vi "IMUOrientOpen.vi"(5 "Stored Cal File":string="BNO055 Cal MC P3 11-28-2015 145653", 7 "Calibrate?":bool, 8 "Status delay":i32=30, 9 "I2C Bus 2":T3=enum."I2C MXP", 10 "Placement":T8(ring)=enum."P3", 11 "Op Mode":T6(ring)=enum."NDOF") -> (0 "Bad result":bool, 2 "Cal Status":T4, 3 "I2CDevRef":T1={"DevStatus"={"status"=FALSE, "code"=0, "source"=""}, "Controller"=enum."Controller 1", "Device Address"=0, "Handle"=0, "I2C Bus"=enum."Invalid"} {"Device Address" format="%.0x"})   [LabVIEW 2014]
uses:
  <vilib>/Rock Robotics/SystemInterfaces/i2clib/i2c_bus.ctl
  Setup State.ctl
  <vilib>/Rock Robotics/WPI/I2C/WPI_I2CDevRef.ctl
  <vilib>/Rock Robotics/SystemInterfaces/Typedef/FPGA_TypedefDigitalModule.ctl
panel:
  out "Bad ct":i32
  out "SC ct":i32
  out "S":T5
  out "G":T5
  out "A":T5
  out "M":T5
  out "Bad result":bool
  out "Fusion":bool
  out "Fusion ct":i32
  out "Reset ct":i32
  out "Occupant":u8[](array[numeric]) format="%02x"
  out "Setup ct":i32
  out "Setup State":T7
  # "Manual Cal\nCalibration Status Indicator"
  # "Diagnostics"
  # "These controls/indicators are non-operational / they are here as example documentation only."
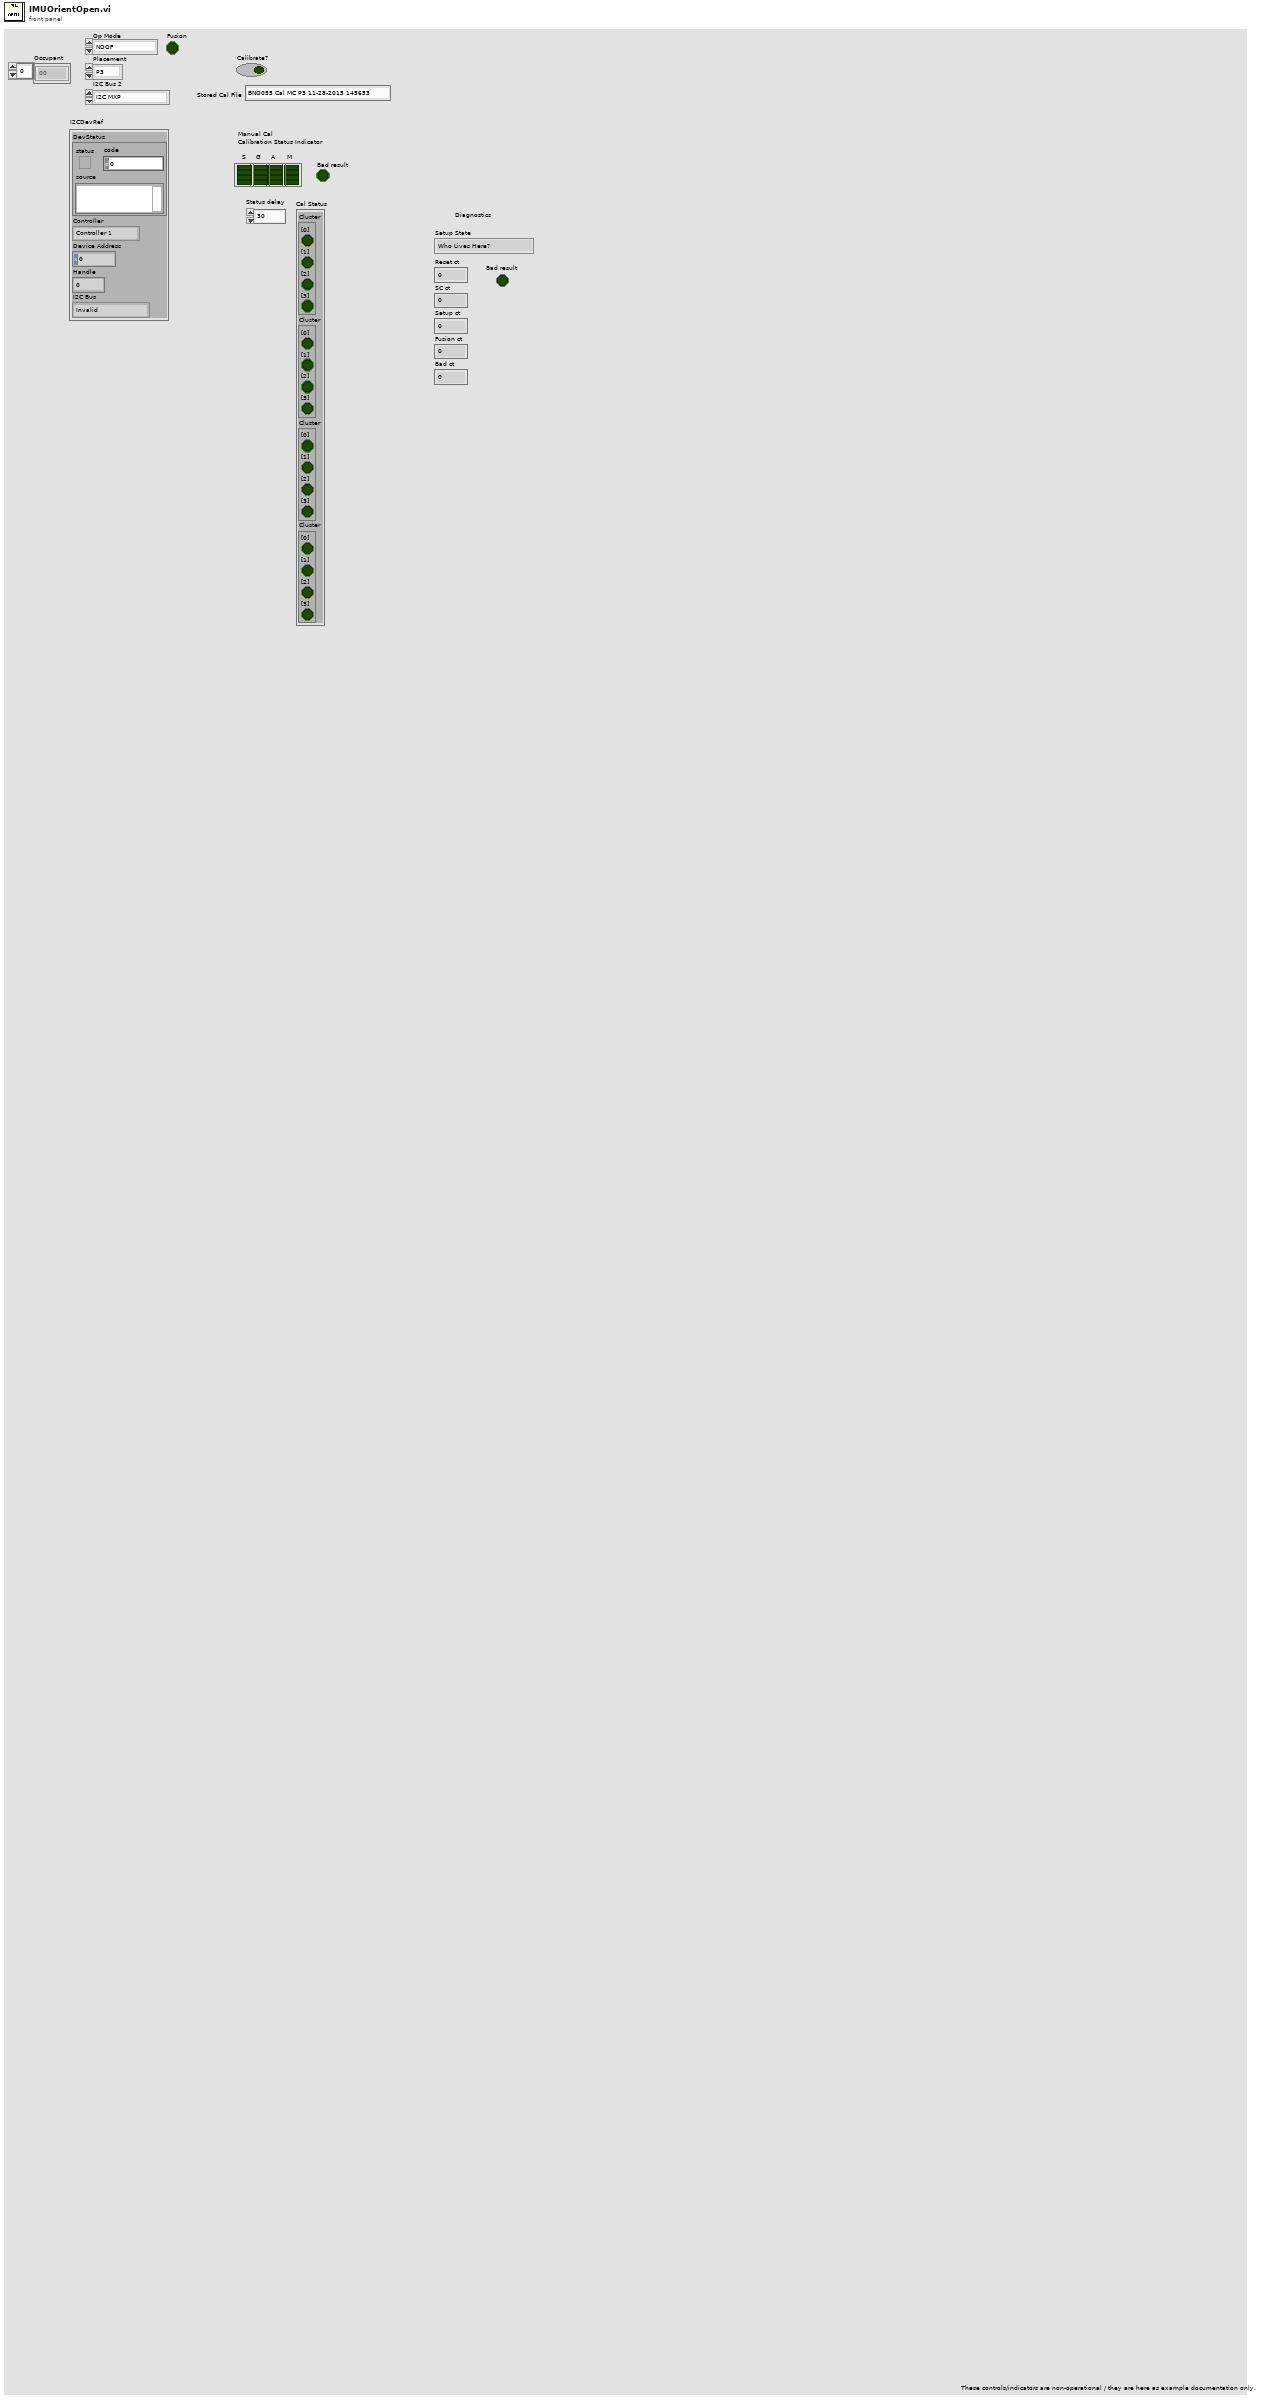
[diagram p1: front panel]
types:
  T1 = typedef "WPI_I2CDevRef.ctl" = cluster{"DevStatus":errorcluster, "Controller":T2, "Device Address":u8, "Handle":i32, "I2C Bus":T3}
  T2 = typedef "FPGA_TypedefDigitalModule.ctl" = enum16{"Controller 1"}
  T3 = typedef "i2c_bus.ctl" = enum16{"I2C On-Board", "I2C MXP", "Invalid"}
  T4 = cluster{"Cluster":cluster{"[0]":bool, "[1]":bool, "[2]":bool, "[3]":bool}, "Cluster":cluster{"[0]":bool, "[1]":bool, "[2]":bool, "[3]":bool}, "Cluster":cluster{"[0]":bool, "[1]":bool, "[2]":bool, "[3]":bool}, "Cluster":cluster{"[0]":bool, "[1]":bool, "[2]":bool, "[3]":bool}}
  T5 = cluster{"Boolean":bool, "Boolean 2":bool, "Boolean 3":bool, "Boolean 4":bool}
  T6 = enum8{"ConfigMode", "AccOnly", "MagOnly", "GyroOnly", "AccMag", "AccGyro", "MagGyro", "AMG", "IMU", "Compass", "M4G", "NDOF_FMC_OFF", "NDOF"}
  T7 = typedef "Setup State.ctl" = enum16{"Who Lives Here?", "Config Mode", "Page 0", "Reset", "Units, Xtal, & Placement", "Fusion Mode", "Pre Calibration", "Error Check", "Manual Cal", "Save Cal", "Restore Cal", "Cal Status", "Idle"}
  T8 = enum32{"P0", "P1", "P2", "P3", "P4", "P5", "P6", "P7"}
  T9 = enum16{"open", "open or create", "create or replace", "create", "open (read-only)"}
  T10 = enum8{"ConfigMode", "AccOnly", "MagOnly", "GyroOnly", "AccMag", "AccGyro", "MagGyro", "AMG", "IMU", "Compass", "M4G", "NDOF_FMC_OFF", "NDOF"}[]
  T11 = cluster{"[0]":bool, "[1]":bool, "[2]":bool, "[3]":bool}
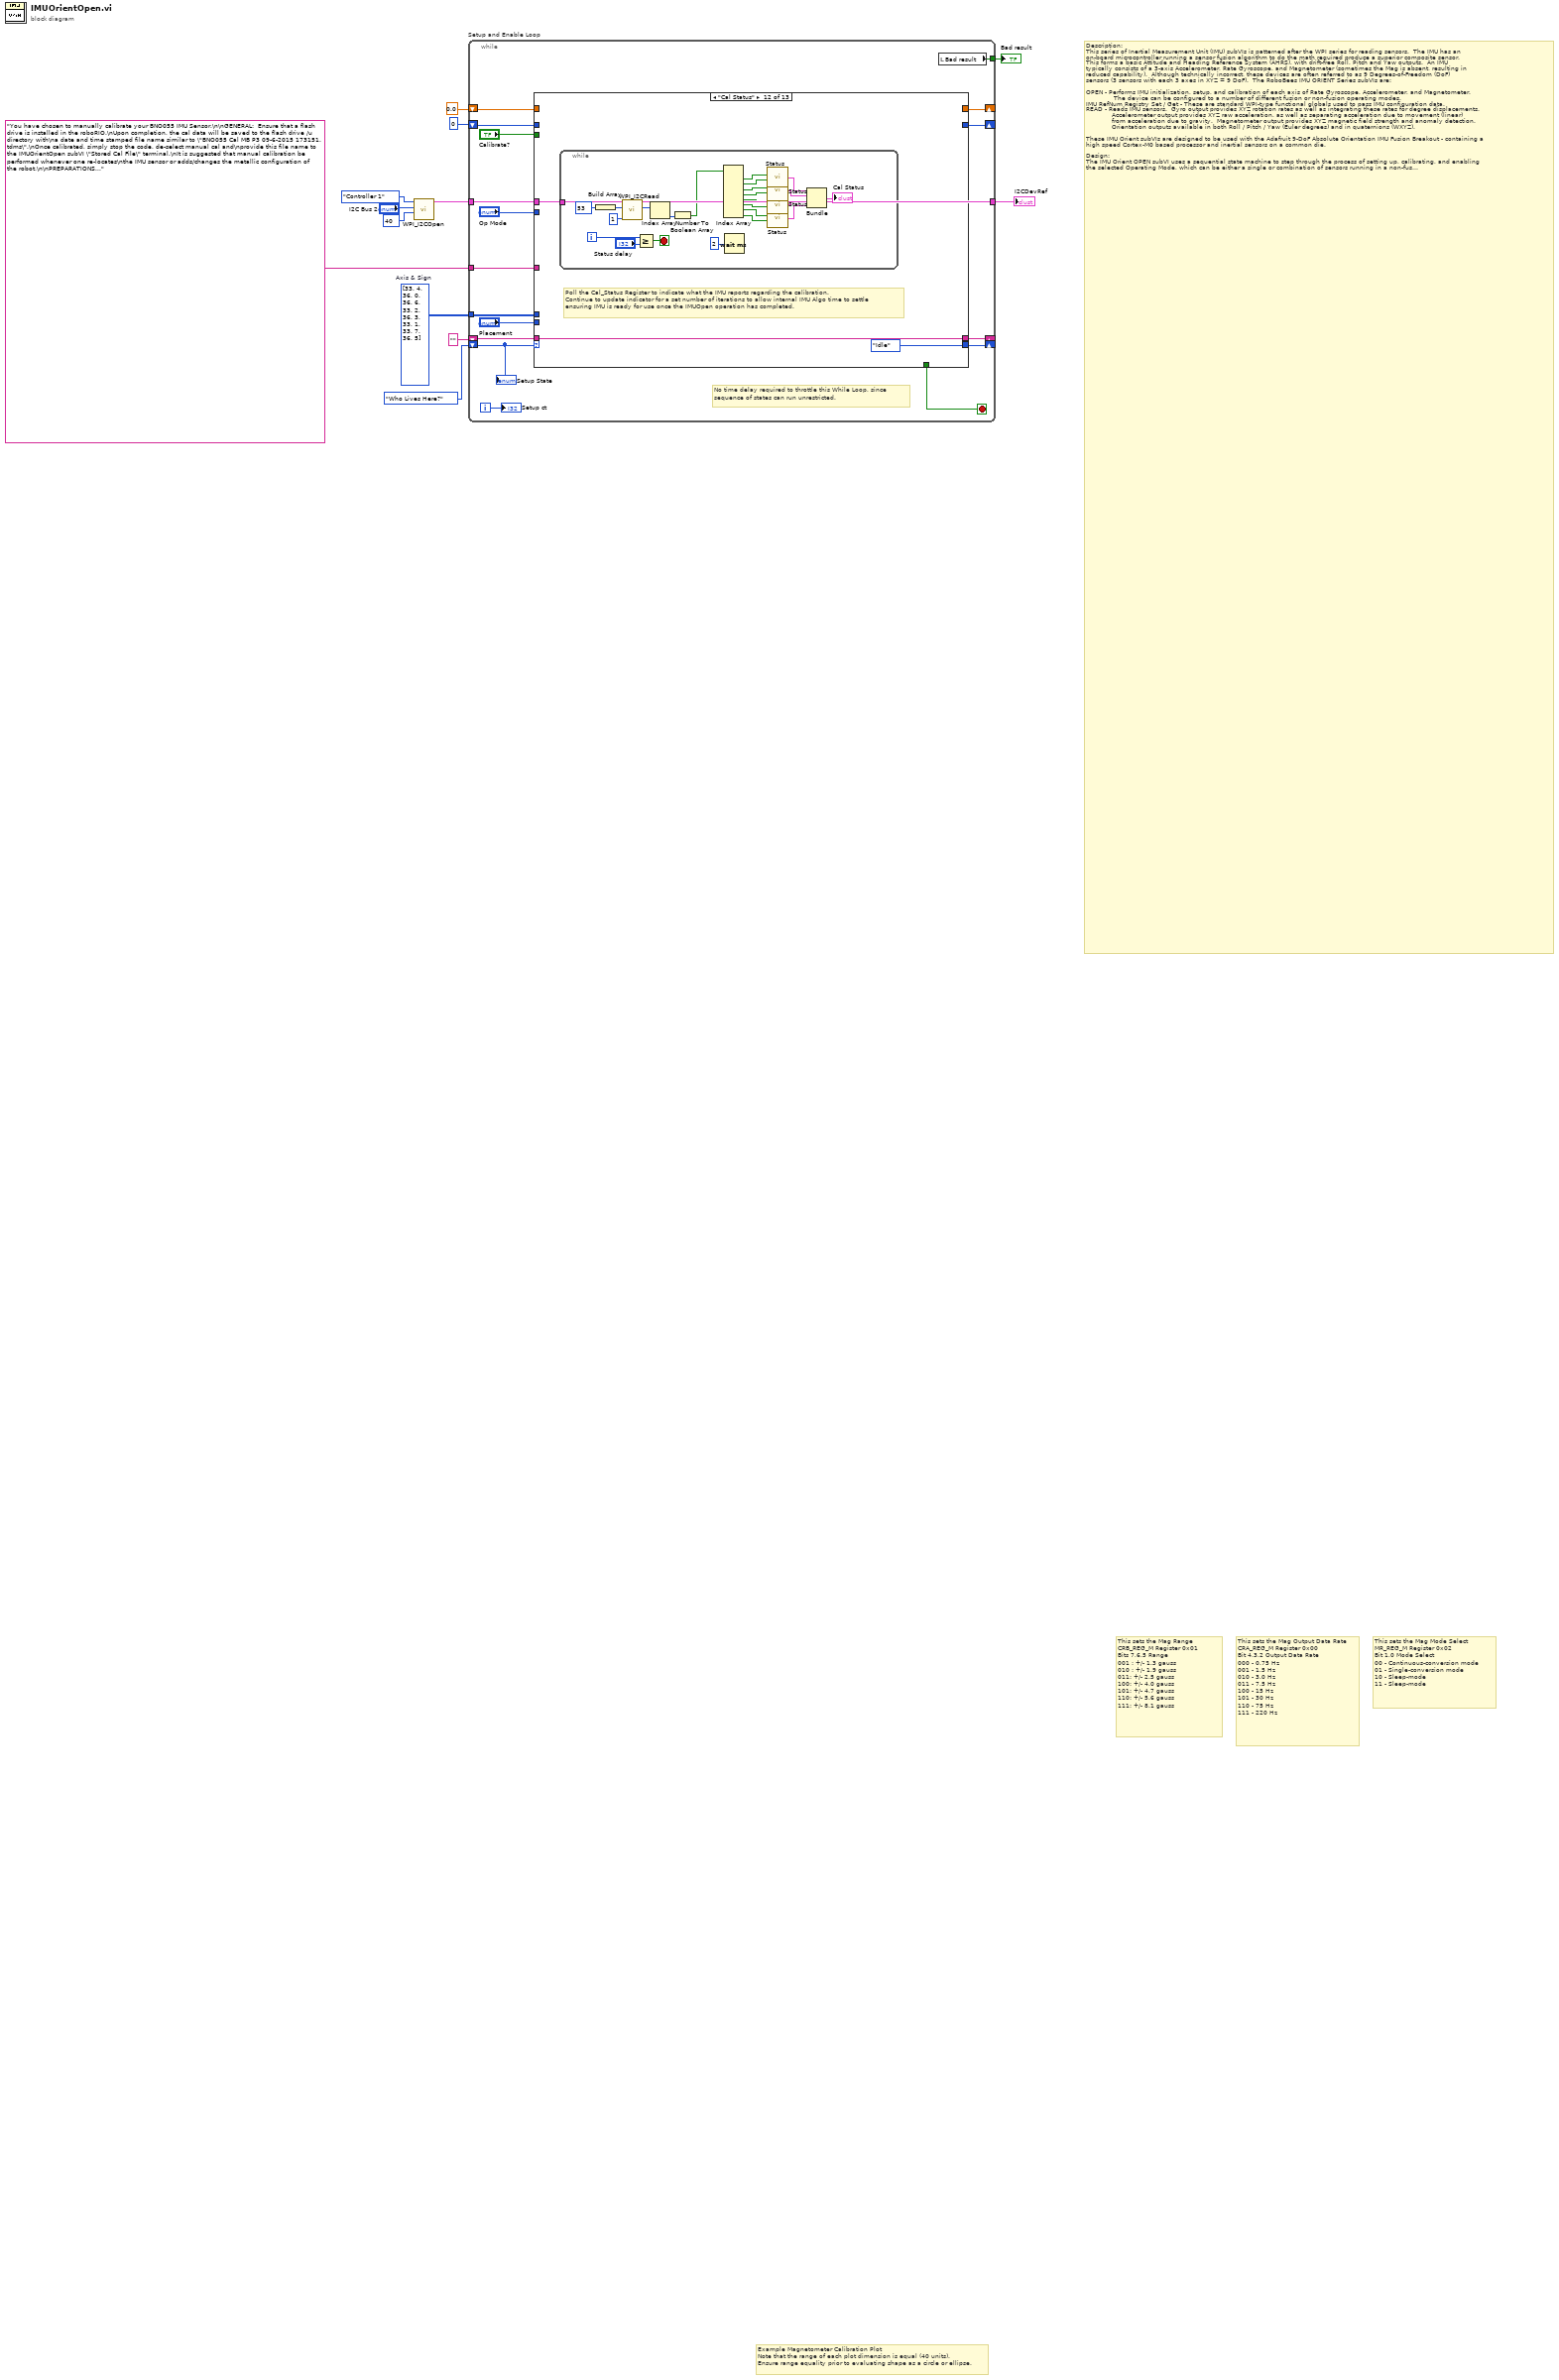
[diagram p0: block diagram]
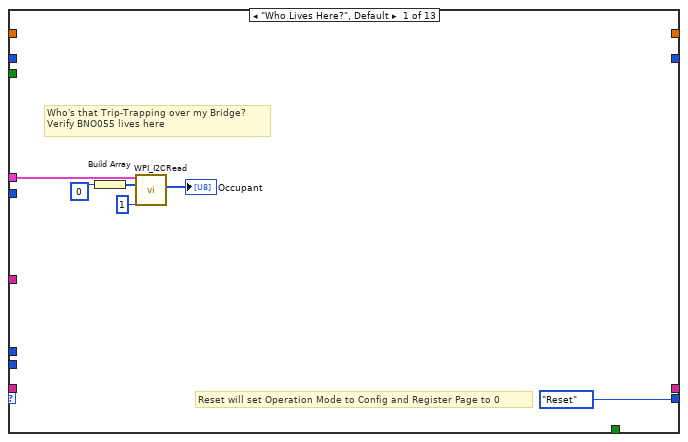
[diagram p2: hidden frame]
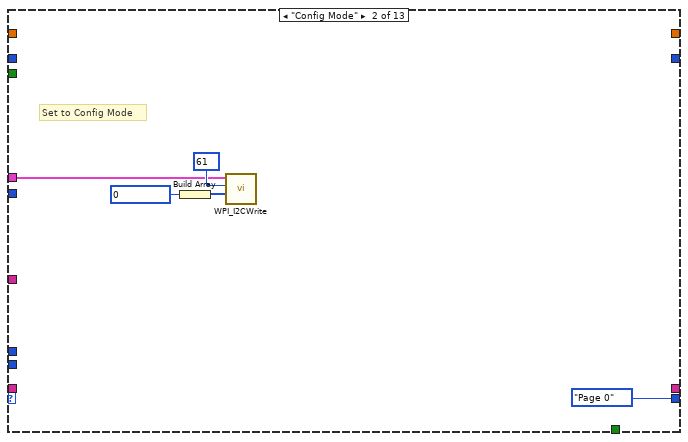
[diagram p3: hidden frame]
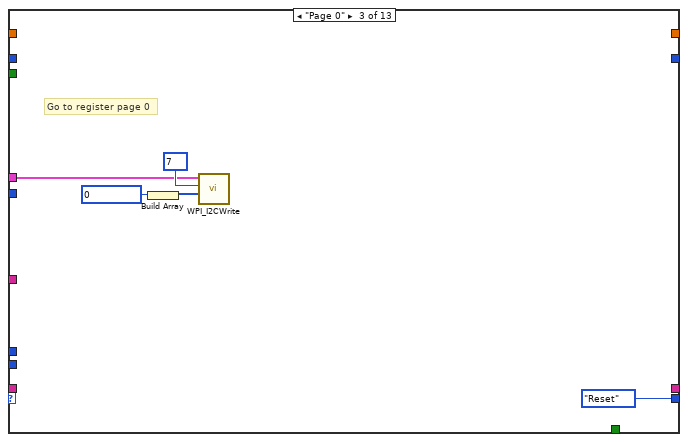
[diagram p4: hidden frame]
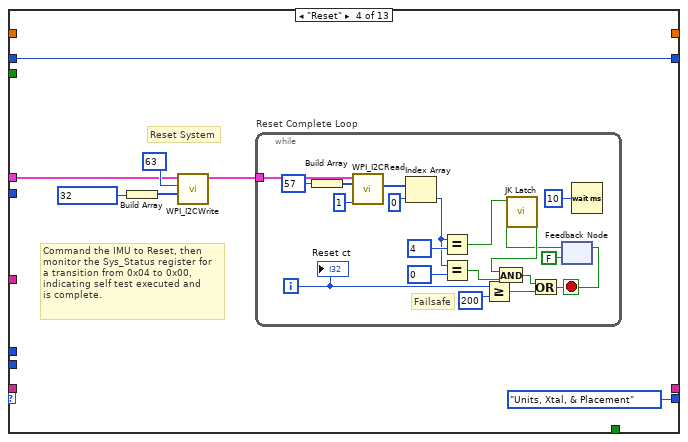
[diagram p5: hidden frame]
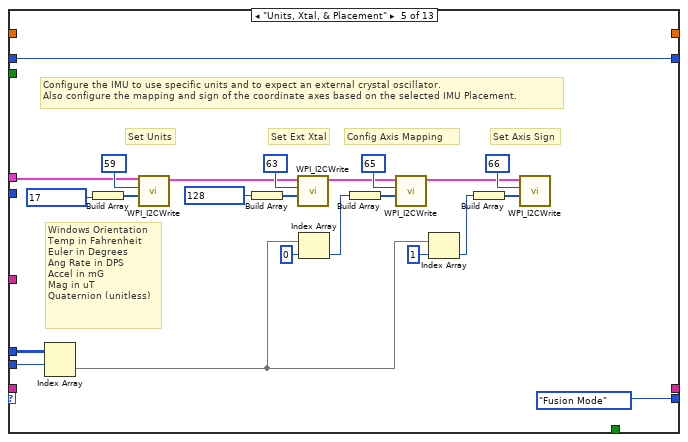
[diagram p6: hidden frame]
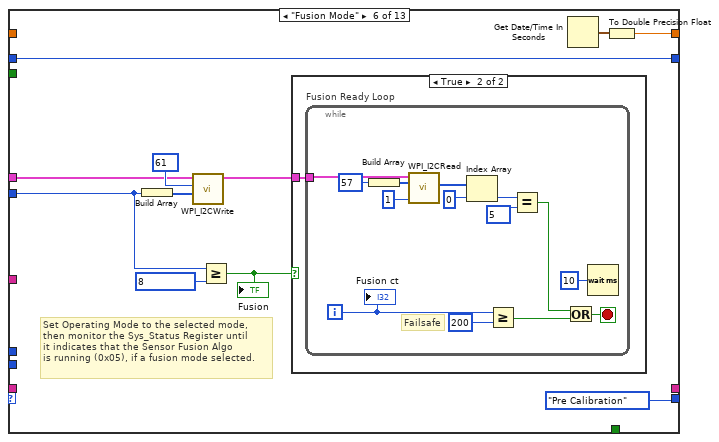
[diagram p7: hidden frame]
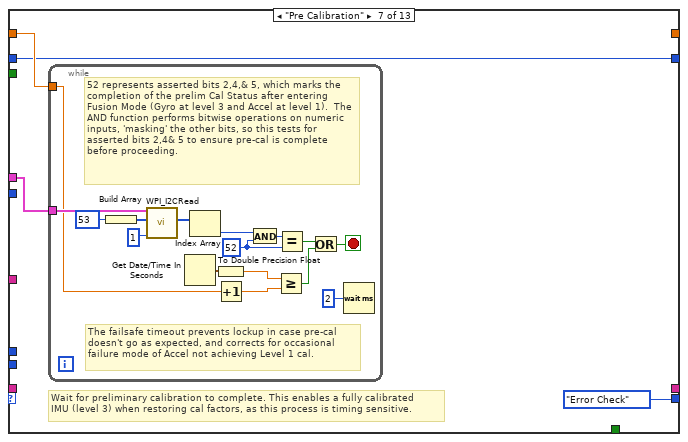
[diagram p9: hidden frame]
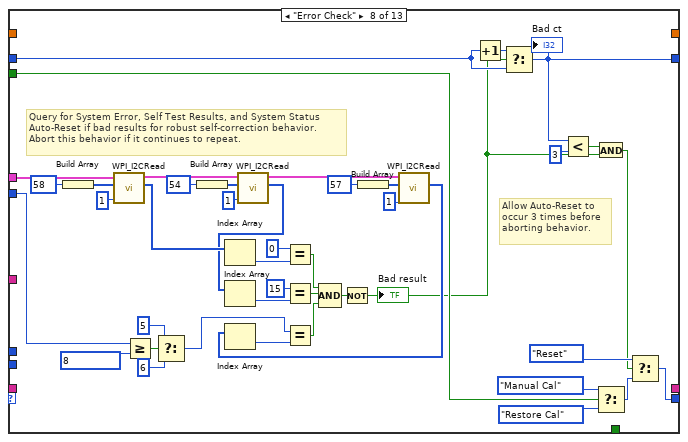
[diagram p10: hidden frame]
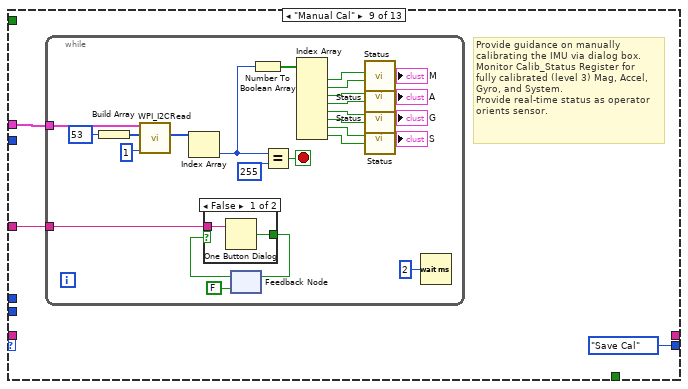
[diagram p11: hidden frame]
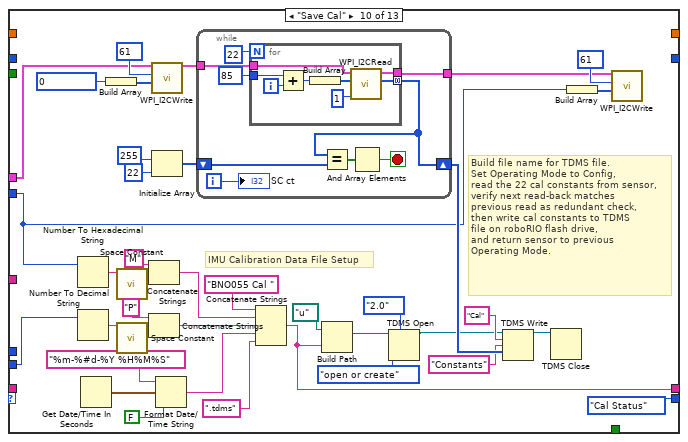
[diagram p13: hidden frame]
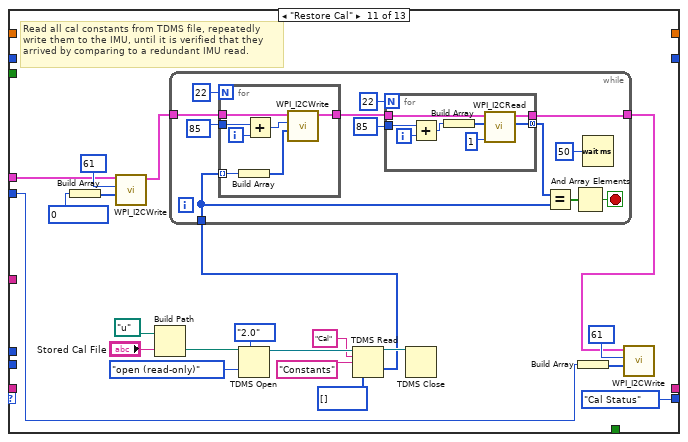
[diagram p14: hidden frame]
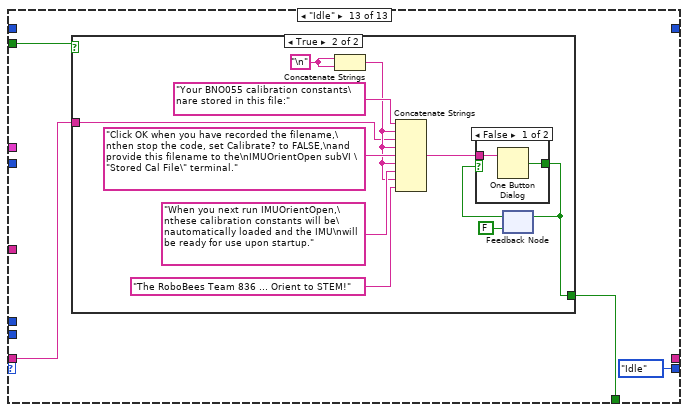
[diagram p15: hidden frame]
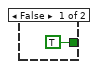
[diagram p16: hidden frame]
diagram:
  w8 = u8[][] [[33, 4], [36, 0], [36, 6], [33, 2], [36, 3], [33, 1], [33, 7], [36, 5]]  # Axis & Sign
  # "Description:\nThis series of Inertial Measurement Unit (IMU) subVIs is patterned after the WPI series for reading sensors.  The IMU has an\non-board microcontroller running a sensor fusion algorithm to do the math required produce a superior composite sensor.\nThis forms a basic Attitude and Heading Reference System (AHRS), with drift-free Roll, Pitch and Yaw outputs.  An IMU\ntypically consists of a 3-axis Accelerometer, Rate Gyroscope, and Magnetometer (sometimes the Mag is absent, resulting in\nreduced capability).  Although technically incorrect, these devices are often referred to as 9 Degrees-of-Freedom (DoF)\nsensors (3 sensors with each 3 axes in XYZ = 9 DoF).  The RoboBees IMU ORIENT Series subVIs are:\n\nOPEN - Performs IMU initialization, setup, and calibration of each axis of Rate Gyroscope, Accelerometer, and Magnetometer.\n              The device can be configured to a number of different fusion or non-fusion operating modes.\nIMU RefNum Registry Set / Get - These are standard WPI-type functional globals used to pass IMU configuration data.\nREAD - Reads IMU sensors.  Gyro output provides XYZ rotation rates as well as integrating these rates for degree displacements.\n             Accelerometer output provides XYZ raw acceleration, as well as separating acceleration due to movement (linear)\n             from acceleration due to gravity.  Magnetometer output provides XYZ magnetic field strength and anomaly detection.\n             Orientation outputs available in both Roll / Pitch / Yaw (Euler degrees) and in quaternions (WXYZ).\n\nThese IMU Orient subVIs are designed to be used with the Adafruit 9-DoF Absolute Orientation IMU Fusion Breakout - containing a\nhigh speed Cortex-M0 based processor and inertial sensors on a common die.\n\nDesign:\nThe IMU Orient OPEN subVI uses a sequential state machine to step through the process of setting up, calibrating, and enabling\nthe selected Operating Mode, which can be either a single or combination of sensors running in a non-fusion mode, or one of\nseveral fusion operating modes.\n\nThe IMU breakout board from Adafruit.com has a single I2C bus for communication.  The sensor I2C Address (in hex) and\nrespective data sheets for I2C register references are:\n\nI2C Address  -  Data Sheet Reference\n       0x28        -  https://ae-bst.resource.bosch.com/media/products/dokumente/bno055/BST_BNO055_DS000_13.pdf\n\nNote: The Adafruit website links to an older version of the BNO055 spec sheet (ver 1.2).  The Bosch site will maintain the latest\nversion.  The link above is the latest revision (ver 1.3) as of January 2016 (released August 2015).   This is a highly sophisticated\nsensor, with many control options, so it is recommended that one review the spec sheet to understand all its capabilities.\n\nSome design effort was expended in an attempt to ensure high reliability of operation.  Data transfer between the sensor cal registers\nand the required flash drive (where cal constants are stored during power down periods) is redundantly verified to be successful.  (Testing\nindicated this to be necessary.)  Upon initialization, if the sensor fails its internal self test, the code will attempt to reset the sensor.\nThis will only occur three times to avoid an infinite loop, which might otherwise prevent a robot from executing operations code.\n\nCalibration:\nRaw readings from an IMU are not very useful until they are conditioned by carefully determined calibration parameters.  One of\nthe key differences between this IMU and others, such as the one discussed here: \n\n                                                         http://www.chiefdelphi.com/forums/showthread.php?t=131823 \n\nis that this BNO055 contains an integrated microcontroller, running a sensor fusion algorithm, which is designed to constantly\nself-calibrate in real-time, after an initial calibration process has occurred.  So, unlike other IMUs that require interface code, this\nIMU really only requires code to trigger the on-board calibration code.  This makes the code for the sensor READ operations simple,\nand the complex code integration requirement associated only with the sensor OPEN (although one only has to trigger the on-board\ncal process, doing this reliably and providing functionality to store/reload the results still drives code sophistication requirements).\n\nOnce the state machine has initialized the sensor, a user-selected control is referenced to either initiate the sensor's embedded\ncal process or read previously stored calibration constants from a file.  [Note: this vi expects a flash drive to be installed in one\nof the roboRIOs USB ports for cal file storage/retrieval].   A dialog box is used to instruct the user on the sensor movements required\nfor calibration, and a Calibration Status Indicator is provided on this vi's front panel to provide feedback and track progress.   Once\ncal is complete, the filename containing the cal constants is displayed.  De-selecting the cal control and providing the cal filename\nto this vi enables the sensor to open in a ready-for-use state.\n\nThe cal filename will contain the Operating Mode, Placement (sensor orientation), and a timestamp to help distinguish one file\nfrom another.  The Op Mode and Placement are included as there is some indication in testing that one should not expect the cal\nto be correct when these parameters differ between cal and use.\n\nVI Properties:\nExecution Reentrancy is set to Non Reentrant Execution\n\nImplementation:\nIt is recommended that the MXP I2C Interface is used, rather than the On-Board I2C Interface, as the latter can generate glitches from\nLo/Hi byte pairing failures when data is reassembled across paired measurement registers.\n\nA visualization vi is provided to observe orientation change as the sensor is moved.  It currently has a bug, causing an error box to\nappear when first run.  Simply click OK and the visualization will occur on the vi's Front Panel.  The vi runs on the My Computer Target,\n(not the roboRIO Target), which means it can only be accessed in debug mode.  There is an issue where Roll exceeding ~45 degrees\ncauses an orientation error.\n \nIt is important to note that while the P/R/Y values are constrained, the Gyro displacement values in X/Y/Z are not.  Gyro deg outputs\nfrom the IMU ORIENT READ subVI will wind (not wrap) - i.e. they will continue to count above/below 360 degrees.  Use the LabVIEW\nQuotient & Remainder (modulus) function to convert these outputs to a wrapping behavior, if desired. \n\nImplementation considerations for IMU Read:\nThis design performs numerical integration off-FPGA for the Digital Gyro (unlike the Analog Gyro subVIs, which typically utilize\nthe FPGA to perform accumulation for superior speed resulting in less integration error).   Testing indicates this off-FPGA\napproach may be adequate for FRC application, however, it is important to ensure the code runs without any timing issues.\nThis is why a Timed Loop is recommended for the IMU Read within Periodic Tasks (executes at a higher priority).  Non-uniformity\nin read iteration is mitigated by design, as each dt is uniquely calculated by time stamping each read event.  This means that while\nsome variation in timing can be tolerated (the occasional late iteration), excessively long durations (periods) between successive\nreads will fail to capture the actual rate profile as it changes resulting in integration error.  \n\nIn short, use a Timed Loop structure to iterate IMU READs, and set the loop period for a relatively fast iteration (<75 ms).  Shorter\nperiods provide improved accuracy of degree displacements, however setting this too short can impact the execution of your\nremaining code (especially when using Timed Loops).  One way of determining an optimized period is to set it while monitoring\nthe \"Finished Late?\" Loop parameter, ensuring this value stays False.   It helps if the CPU Utilization remains low (<75%), which\ncan be monitored with the RT Get CPU Loads subVI (Real Time menu).  Study LabVIEW determinism for additional insight.\n\n----- RoboBees FRC Team 836! -----  You too can conquer inertia!! ... ORIENT on a career in STEM!"
  # "Example Magnetometer Calibration Plot\nNote that the range of each plot dimension is equal (40 units).\nEnsure range equality prior to evaluating shape as a circle or ellipse."
  # "This sets the Mag Mode Select\nMR_REG_M Register 0x02\nBit 1,0 Mode Select\n00 - Continuous-conversion mode \n01 - Single-conversion mode\n10 - Sleep-mode\n11 - Sleep-mode"
  # "This sets the Mag Output Data Rate\nCRA_REG_M Register 0x00\nBit 4,3,2 Output Data Rate\n000 - 0.75 Hz \n001 - 1.5 Hz \n010 - 3.0 Hz\n011 - 7.5 Hz\n100 - 15 Hz\n101 - 30 Hz\n110 - 75 Hz\n111 - 220 Hz"
  # "This sets the Mag Range\nCRB_REG_M Register 0x01\nBits 7,6,5 Range\n001 : +/- 1.3 gauss\n010 : +/- 1.9 gauss\n011: +/- 2.5 gauss\n100: +/- 4.0 gauss\n101: +/- 4.7 gauss\n110: +/- 5.6 gauss\n111: +/- 8.1 gauss"
  n1 = call <vilib>:"WPI_I2COpen.vi"("Device Address"=u8 40, "I2C Bus"="I2C Bus 2", "Controller"=FPGA_TypedefDigitalModule."Controller 1" ("Controller 2")) -> ("I2CDevRef"=w9:T1)  [unwired: 7 in, 1 out]
  n2 = while "Setup and Enable Loop" {
    tunnel: w9 -> [w23]
    tunnel: "You have chosen to manually calibrate your BNO055 IMU Sensor.\n\nGENERAL:  Ensure that a flash drive is installed in the roboRIO.\nUpon completion, the cal data will be saved to the flash drive /u directory with\na date and time stamped file name similar to \"BNO055 Cal MB P3 09-6-2015 173151.tdms\".\nOnce calibrated, simply stop the code, de-select manual cal and\nprovide this file name to the IMUOrientOpen subVI \"Stored Cal File\" terminal.\nIt is suggested that manual calibration be performed whenever one re-locates\nthe IMU sensor or adds/changes the metallic configuration of the robot.\n\nPREPARATIONS:  If sensor is installed on a robot, ensure sensor is secure.\nThese device movement instructions will then apply to entire robot.\nAs you proceed, monitor the Calibration Status Indicator on the IMUOrientOpen Front Panel.\nCalibration is complete when all indicators are Green.\n\nGYRO CAL:  Allow device to maintain a single stable\nposition to enable Gyro to self-calibrate.\n\nACCELEROMETER CAL:  Place device in 6 different stable\npositions for a few seconds to allow it to calibrate.\nEnsure there is slow movement between 2 stable positions.\nThe 6 stable positions can be in any direction, but ensure the\ndevice is perpendicular to the X,Y & Z axis at least once.\nThis is usually the most difficult device to calibrate.\nIf problematic, try slowing down the movement between positions.\n\nMAGNETOMETER CAL:  Make random movements\nin all 3 axes until Cal Status Indicator is Green.\n\nSYSTEM CAL:  Alternately move device and hold still until\nCal Status Indicator is Green, if necessary. \n\nClick OK when ready to begin." ("message") -> [w28]
    tunnel: w8 -> [w26]
    tunnel: [w23] -> w7
    shift-right: [w21] -> _
    shift-left: 0 -> [w20]
    tunnel: [w19] -> w4
    shift-right: [w18] -> _
    shift-left: 0.0 -> [w17]
    shift-right: [w16] -> _
    shift-left: "" -> [w15]
    shift-right: [w14] -> _
    shift-left: Setup_State."Who Lives Here?" -> [w13]
    i -> [w25]
    stop <- w24 stop-if-true
    # "No time delay required to throttle this While Loop, since sequence of states can run unrestricted."
    n3 = case shown="\"Cal Status\"" w13 {
      tunnel: [Setup_State."Reset" Setup_State."Page 0" Setup_State."Reset" Setup_State."Units, Xtal, & Placement" Setup_State."Fusion Mode" Setup_State."Pre Calibration" Setup_State."Error Check" w157 Setup_State."Save Cal" Setup_State."Cal Status" Setup_State."Cal Status" Setup_State."Idle" Setup_State."Idle"] -> w14
      tunnel: w23 -> [w32 w36 w42 w49 w87 w104 w125 w173 w187 w248 w277 w322 _]
      tunnel: "Calibrate?" -> [_ _ _ _ _ _ _ w145 _ _ _ _ w350]
      tunnel: [_ _ _ _ _ w101 _ _ _ _ _ _ _] -> w18
      tunnel: w17 -> [_ _ _ _ _ _ w123 _ _ _ _ _ _]
      tunnel: w28 -> [_ _ _ _ _ _ _ _ w185 _ _ _ _]
      tunnel: "Placement" -> [_ _ _ _ w77 _ _ _ _ w221 _ _ _]
      tunnel: w26 -> [_ _ _ _ w75 _ _ _ _ _ _ _ _]
      tunnel: [_ _ _ _ _ _ _ _ _ w218 _ w320 _] -> w16
      tunnel: [_ _ _ _ _ _ _ _ _ _ _ _ w349] -> w24
      tunnel: w15 -> [_ _ _ _ _ _ _ _ _ _ _ w320 w348]
      tunnel: "Op Mode" -> [_ _ _ _ _ w97 _ w150 _ w217 w272 _ _]
      tunnel: [_ _ _ w46 w73 w96 w122 w147 _ _ _ _ _] -> w21
      tunnel: w20 -> [_ _ _ w46 w73 w96 w122 w148 _ _ _ _ _]
      frame "Who Lives Here?", Default {
        # "Reset will set Operation Mode to Config and Register Page to 0"
        # "Who's that Trip-Trapping over my Bridge?\nVerify BNO055 lives here"
        n4 = Build Array(u8 0 ("Data To Send")) -> (w35:u8[])
        n5 = call <vilib>:"WPI_I2CRead.vi"("I2CBytesToRead"=u8 1, "I2CRegister"=w35, "I2CDevRef"=w32) -> ("Data Out"=→"Occupant":u8[])  [unwired: 6 in, 2 out]
      }
      frame "Config Mode" {
        # "Set to Config Mode"
        n6 = Build Array(u8 0 ("I2CRegister")) -> (w40:u8[])
        n7 = call <vilib>:"WPI_I2CWrite.vi"("I2CDataToSend"=w40, "I2CRegister"=u8 61 ("Data To Send hex 2"), "I2CDevRef"=w36) -> ()  [unwired: 7 in, 2 out]
      }
      frame "Page 0" {
        # "Go to register page 0"
        n8 = Build Array(u8 0 ("I2CRegister")) -> (w45:u8[])
        n9 = call <vilib>:"WPI_I2CWrite.vi"("I2CDataToSend"=w45, "I2CRegister"=u8 7 ("Data To Send hex 2"), "I2CDevRef"=w42) -> ()  [unwired: 7 in, 2 out]
      }
      frame "Reset" {
        # "Command the IMU to Reset, then\nmonitor the Sys_Status register for\na transition from 0x04 to 0x00,\nindicating self test executed and\nis complete."
        # "Reset System"
        n10 = Build Array(u8 32 ("I2CRegister")) -> (w52:u8[])
        n11 = call <vilib>:"WPI_I2CWrite.vi"("I2CDataToSend"=w52, "I2CRegister"=u8 63 ("Data To Send hex 2"), "I2CDevRef"=w49) -> ("I2CDevRef"=w47:T1)  [unwired: 7 in, 1 out]
        n12 = while "Reset Complete Loop" {
          tunnel: w47 -> [w67]
          i -> [w55]
          stop <- w57 stop-if-true
          # "Failsafe"
          n13 = Build Array(u8 57 ("Data To Send")) -> (w70:u8[])
          n14 = call <vilib>:"WPI_I2CRead.vi"("I2CBytesToRead"=u8 1, "I2CRegister"=w70, "I2CDevRef"=w67) -> ("Data Out"=w69:u8[])  [unwired: 6 in, 2 out]
          n15 = Index Array(array=w69, index=0 ("disabled index (col)")) -> (element=w56:u8)
          n16 = Equal?(x=w56, y=u8 4 ("I2CBytesToRead")) -> (x = y?=w62:bool)
          n17 = Equal?(x=w56, y=u8 0 ("I2CBytesToRead")) -> (x = y?=w61:bool)
          n18 = Greater Or Equal?(x=w55, y=200) -> (x >= y?=w59:bool)
          n19 = feedback #1(FALSE) -> (w54:bool)
          n20 = call <userlib>:"JK Latch.vi"("Reset"=w54, "Set"=w62) -> ("Q"=w63:bool)  [unwired: 5 in]
          n21 = And(x=w63, y=w61) -> (x .and. y?=w60:bool)
          n22 = Or(x=w60, y=w59) -> (x .or. y?=w57:bool)
          n23 = feedback-in #1(w57) -> ()
          n24 = Wait (ms)(milliseconds to wait=u32 10) -> ()  [unwired: 1 out]
          "Reset ct" <- w55
        }
      }
      frame "Units, Xtal, & Placement" {
        # "Configure the IMU to use specific units and to expect an external crystal oscillator.\nAlso configure the mapping and sign of the coordinate axes based on the selected IMU Placement."
        # "Set Axis Sign"
        # "Config Axis Mapping"
        # "Set Ext Xtal"
        # "Windows Orientation\nTemp in Fahrenheit\nEuler in Degrees\nAng Rate in DPS\nAccel in mG\nMag in uT\nQuaternion (unitless)"
        # "Set Units"
        n25 = Index Array(array=w75, index (row)=w77) -> (element=w78:u8[])  [unwired: 1 in]
        n26 = Build Array(u8 17 ("I2CRegister")) -> (w95:u8[])
        n27 = call <vilib>:"WPI_I2CWrite.vi"("I2CDataToSend"=w95, "I2CRegister"=u8 59 ("Data To Send hex 2"), "I2CDevRef"=w87) -> ("I2CDevRef"=w89:T1)  [unwired: 7 in, 1 out]
        n28 = Build Array(u8 128 ("I2CRegister")) -> (w94:u8[])
        n29 = call <vilib>:"WPI_I2CWrite.vi"("I2CDataToSend"=w94, "I2CRegister"=u8 63 ("Data To Send hex 2"), "I2CDevRef"=w89) -> ("I2CDevRef"=w84:T1)  [unwired: 7 in, 1 out]
        n30 = Index Array(array=w78, index=0) -> (element=w76:u8)
        n31 = Build Array(w76) -> (w85:u8[])
        n32 = call <vilib>:"WPI_I2CWrite.vi"("I2CDataToSend"=w85, "I2CRegister"=u8 65 ("Data To Send hex 2"), "I2CDevRef"=w84) -> ("I2CDevRef"=w81:T1)  [unwired: 7 in, 1 out]
        n33 = Index Array(array=w78, index=1) -> (element=w74:u8)
        n34 = Build Array(w74) -> (w83:u8[])
        n35 = call <vilib>:"WPI_I2CWrite.vi"("I2CDataToSend"=w83, "I2CRegister"=u8 66 ("Data To Send hex 2"), "I2CDevRef"=w81) -> ()  [unwired: 7 in, 2 out]
      }
      frame "Fusion Mode" {
        # "Set Operating Mode to the selected mode,\nthen monitor the Sys_Status Register until\nit indicates that the Sensor Fusion Algo\nis running (0x05), if a fusion mode selected."
        n36 = Build Array(w97) -> (w106:T10)
        n37 = call <vilib>:"WPI_I2CWrite.vi"("I2CDataToSend"=w106, "I2CRegister"=u8 61 ("Data To Send hex 2"), "I2CDevRef"=w104) -> ("I2CDevRef"=w103:T1)  [unwired: 7 in, 1 out]
        n38 = Greater Or Equal?(x=w97, y=u8 8 ("I2CRegister")) -> (x >= y?=w99:bool)
        "Fusion" <- w99
        n39 = case shown="True" w99 {
          tunnel: w103 -> [_ w107]
          frame False {
          }
          frame True {
            n40 = while "Fusion Ready Loop" {
              tunnel: w107 -> [w116]
              i -> [w111]
              stop <- w115 stop-if-true
              # "Failsafe"
              n41 = Build Array(u8 57 ("Data To Send")) -> (w119:u8[])
              n42 = call <vilib>:"WPI_I2CRead.vi"("I2CBytesToRead"=u8 1, "I2CRegister"=w119, "I2CDevRef"=w116) -> ("Data Out"=w118:u8[])  [unwired: 6 in, 2 out]
              n43 = Index Array(array=w118, index=0 ("disabled index (col)")) -> (element=w108:u8)
              n44 = Greater Or Equal?(x=w111, y=200) -> (x >= y?=w112:bool)
              n45 = Equal?(x=w108, y=u8 5 ("I2CBytesToRead")) -> (x = y?=w114:bool)
              n46 = Or(x=w114, y=w112) -> (x .or. y?=w115:bool)
              n47 = Wait (ms)(milliseconds to wait=u32 10) -> ()  [unwired: 1 out]
              "Fusion ct" <- w111
            }
          }
        }
        n48 = Get Date/Time In Seconds() -> (seconds since 1Jan1904=w102:timestamp)
        n49 = To Double Precision Float(number=w102) -> (double precision float=w101:dbl)
      }
      frame "Pre Calibration" {
        # "Wait for preliminary calibration to complete. This enables a fully calibrated\nIMU (level 3) when restoring cal factors, as this process is timing sensitive."
        n50 = while {
          tunnel: w125 -> [w137]
          tunnel: w123 -> [w127]
          stop <- w132 stop-if-true
          w133 = u8 52 ("y")
          # "The failsafe timeout prevents lockup in case pre-cal\ndoesn't go as expected, and corrects for occasional\nfailure mode of Accel not achieving Level 1 cal."
          # "52 represents asserted bits 2,4,& 5, which marks the completion of the prelim Cal Status after entering Fusion Mode (Gyro at level 3 and Accel at level 1).  The AND function performs bitwise operations on numeric inputs, 'masking' the other bits, so this tests for asserted bits 2,4& 5 to ensure pre-cal is complete before proceeding."
          n51 = Build Array(u8 53 ("Data To Send")) -> (w141:u8[])
          n52 = call <vilib>:"WPI_I2CRead.vi"("I2CBytesToRead"=u8 1, "I2CRegister"=w141, "I2CDevRef"=w137) -> ("Data Out"=w138:u8[])  [unwired: 6 in, 2 out]
          n53 = Get Date/Time In Seconds() -> (seconds since 1Jan1904=w131:timestamp)
          n54 = Index Array(array=w138) -> (element=w134:u8)  [unwired: 1 in]
          n55 = To Double Precision Float(number=w131) -> (double precision float=w128:dbl)
          n56 = Increment(x=w127) -> (x+1=w126:dbl)
          n57 = And(x=w134, y=w133) -> (x .and. y?=w135:u8)
          n58 = Greater Or Equal?(x=w128, y=w126) -> (x >= y?=w129:bool)
          n59 = Equal?(x=w135, y=w133) -> (x = y?=w130:bool)
          n60 = Or(x=w130, y=w129) -> (x .or. y?=w132:bool)
          n61 = Wait (ms)(milliseconds to wait=u32 2 ("pre-cal wait")) -> ()  [unwired: 1 out]
        }
      }
      frame "Error Check" {
        # "Allow Auto-Reset to\noccur 3 times before\naborting behavior."
        # "Query for System Error, Self Test Results, and System Status\nAuto-Reset if bad results for robust self-correction behavior.\nAbort this behavior if it continues to repeat."
        n62 = Build Array(u8 58 ("Data To Send")) -> (w182:u8[])
        n63 = call <vilib>:"WPI_I2CRead.vi"("I2CBytesToRead"=u8 1, "I2CRegister"=w182, "I2CDevRef"=w173) -> ("Data Out"=w164:u8[], "I2CDevRef"=w175:T1)  [unwired: 6 in, 1 out]
        n64 = Greater Or Equal?(x=w150, y=u8 8 ("I2CRegister")) -> (x >= y?=w155:bool)
        n65 = Select(t=u8 5 ("x"), s=w155, f=u8 6 ("x")) -> (s? t:f=w152:u8)
        n66 = Build Array(u8 54 ("Data To Send")) -> (w181:u8[])
        n67 = Index Array(array=w164) -> (element=w165:u8)  [unwired: 1 in]
        n68 = call <vilib>:"WPI_I2CRead.vi"("I2CBytesToRead"=u8 1, "I2CRegister"=w181, "I2CDevRef"=w175) -> ("Data Out"=w163:u8[], "I2CDevRef"=w174:T1)  [unwired: 6 in, 1 out]
        n69 = Index Array(array=w163) -> (element=w166:u8)  [unwired: 1 in]
        n70 = Equal?(x=u8 0, y=w165) -> (x = y?=w169:bool)
        n71 = Equal?(x=u8 15, y=w166) -> (x = y?=w170:bool)
        n72 = Build Array(u8 57 ("Data To Send")) -> (w176:u8[])
        n73 = call <vilib>:"WPI_I2CRead.vi"("I2CBytesToRead"=u8 1, "I2CRegister"=w176, "I2CDevRef"=w174) -> ("Data Out"=w162:u8[])  [unwired: 6 in, 2 out]
        n74 = Index Array(array=w162) -> (element=w168:u8)  [unwired: 1 in]
        n75 = Equal?(x=w152, y=w168) -> (x = y?=w171:bool)
        n76 = Compound Arithmetic op=AND(w169, w170, w171) -> (w172:bool)
        n77 = Not(x=w172) -> (.not. x?=w143:bool)
        "Bad result" <- w143
        n78 = Increment(x=w148) -> (x+1=w149:i32)
        n79 = Select(t=w149, s=w143, f=w148) -> (s? t:f=w147:i32)
        "Bad ct" <- w147
        n80 = Less?(x=w147, y=3) -> (x < y?=w142:bool)
        n81 = And(x=w142, y=w143) -> (x .and. y?=w144:bool)
        n82 = Select(t=Setup_State."Manual Cal", s=w145, f=Setup_State."Restore Cal") -> (s? t:f=w158:T7)
        n83 = Select(t=Setup_State."Reset", s=w144, f=w158) -> (s? t:f=w157:T7)
      }
      frame "Manual Cal" {
        # "Provide guidance on manually\ncalibrating the IMU via dialog box.\nMonitor Calib_Status Register for\nfully calibrated (level 3) Mag, Accel,\nGyro, and System. \nProvide real-time status as operator\norients sensor."
        n84 = while {
          tunnel: w187 -> [w209]
          tunnel: w185 -> [w190]
          stop <- w188 stop-if-true
          n85 = Build Array(u8 53 ("Data To Send")) -> (w213:u8[])
          n86 = call <vilib>:"WPI_I2CRead.vi"("I2CBytesToRead"=u8 1, "I2CRegister"=w213, "I2CDevRef"=w209) -> ("Data Out"=w210:u8[])  [unwired: 6 in, 2 out]
          n87 = Index Array(array=w210) -> (element=w194:u8)  [unwired: 1 in]
          n88 = feedback #2(FALSE ("true")) -> (w192:bool)
          n89 = case shown="False" w192 {
            selector: w192 -> [_ w216]
            tunnel: [w215 w216] -> w193
            tunnel: w190 -> [w214 _]
            frame False {
              n90 = One Button Dialog(message=w214) -> (true=w215:bool)  [unwired: 1 in]
            }
            frame True {
            }
          }
          n91 = feedback-in #2(w193) -> ()
          n92 = Number To Boolean Array(number=w194) -> (Boolean array=w195:bool[])
          n93 = Equal?(x=w194, y=u8 255) -> (x = y?=w188:bool)
          n94 = Index Array(array=w195) -> (element #1=w207:bool, element #2=w206:bool, element #3=w205:bool, element #4=w204:bool, element #5=w203:bool, element #6=w202:bool, element #7=w201:bool, element #8=w200:bool)  [unwired: 8 in]
          n95 = call "Status.vi"("Big"=w206, "Little"=w207) -> ("Cluster"=→"M":T11)  [unwired: 2 in]
          n96 = call "Status.vi"("Big"=w204, "Little"=w205) -> ("Cluster"=→"A":T11)  [unwired: 2 in]
          n97 = call "Status.vi"("Big"=w202, "Little"=w203) -> ("Cluster"=→"G":T11)  [unwired: 2 in]
          n98 = call "Status.vi"("Big"=w200, "Little"=w201) -> ("Cluster"=→"S":T11)  [unwired: 2 in]
          n99 = Wait (ms)(milliseconds to wait=u32 2 ("pre-cal wait")) -> ()  [unwired: 1 out]
        }
      }
      frame "Save Cal" {
        # "Build file name for TDMS file.\nSet Operating Mode to Config,\nread the 22 cal constants from sensor,\nverify next read-back matches\nprevious read as redundant check,\nthen write cal constants to TDMS\nfile on roboRIO flash drive,\nand return sensor to previous\nOperating Mode."
        # "IMU Calibration Data File Setup"
        n100 = Number To Hexadecimal String(2:w217) -> (0:w224:string)  [unwired: 1 in]
        n101 = Number To Decimal String(number=w221) -> (decimal integer string=w228:string)  [unwired: 1 in]
        n102 = Get Date/Time In Seconds() -> (seconds since 1Jan1904=w233:timestamp)
        n103 = Build Array(u8 0 ("I2CRegister")) -> (w252:u8[])
        n104 = call <vilib>:"Space Constant.vi"() -> ("String"=w226:string)
        n105 = call <vilib>:"Space Constant.vi"() -> ("String"=w227:string)
        n106 = Concatenate Strings("M" ("string"), w224, w226) -> (w223:string)
        n107 = Concatenate Strings("P" ("string"), w228, w227) -> (w222:string)
        n108 = call <vilib>:"WPI_I2CWrite.vi"("I2CDataToSend"=w252, "I2CRegister"=u8 61 ("Data To Send hex 2"), "I2CDevRef"=w248) -> ("I2CDevRef"=w247:T1)  [unwired: 7 in, 1 out]
        n109 = Initialize Array(u8 255, 22 ("dimension size")) -> (w240:u8[])
        n110 = Format Date/Time String(time format string (%c)="%m-%#d-%Y %H%M%S", seconds (now)=w233, UTC format=FALSE) -> (date/time string=w230:string)
        n111 = while {
          tunnel: w247 -> [w258]
          shift-right: [w255] -> w244
          shift-left: w240 -> [w261]
          tunnel: [w259] -> w245
          i -> [w257]
          stop <- w260 stop-if-true
          n112 = for {
            N: 22 -> [_]
            tunnel: u8 85 ("Data To Send 2") -> [w268]
            tunnel: [w266] -> w255 mode=concatenating
            tunnel: w258 -> [w265]
            tunnel: [w264] -> w259
            i -> [w267]
            n113 = Add(x=w268, y=w267) -> (x+y=w269:i32)
            n114 = Build Array(w269) -> (w270:i32[])
            n115 = call <vilib>:"WPI_I2CRead.vi"("I2CBytesToRead"=u8 1, "I2CRegister"=w270, "I2CDevRef"=w265) -> ("Data Out"=w266:u8[], "I2CDevRef"=w264:T1)  [unwired: 6 in, 1 out]
          }
          n116 = Equal?(x=w255, y=w261) -> (x = y?=w256:bool[])
          n117 = And Array Elements(Boolean array=w256) -> (logical AND=w260:bool)
          "SC ct" <- w257
        }
        n118 = Concatenate Strings("BNO055 Cal " ("string"), w223, w222, w230, ".tdms" ("string")) -> (w218:string)
        n119 = Build Path(base path=path "u:/" ("file path (dialog if empty)"), name or relative path=w218) -> (appended path=w237:path)
        n120 = TDMS Open(7:enum16{"1.0", "2.0"}."2.0" ("file format version (2.0)"), 10:T9."open or create" ("operation (0:open)"), 11:w237) -> (3:w220:refnum<k34>)  [unwired: 4 in, 1 out]
        n121 = TDMS Write(0:w220, 5:"Cal" ("group name in (Untitled)"), 7:"Constants" ("channel name(s) in"), 9:w244) -> (4:w219:refnum<k34>)  [unwired: 2 in, 3 out]
        n122 = TDMS Close(11:w219) -> ()  [unwired: 1 in, 2 out]
        n123 = Build Array(w217) -> (w254:T10)
        n124 = call <vilib>:"WPI_I2CWrite.vi"("I2CDataToSend"=w254, "I2CRegister"=u8 61 ("Data To Send hex 2"), "I2CDevRef"=w245) -> ()  [unwired: 7 in, 2 out]
      }
      frame "Restore Cal" {
        # "Read all cal constants from TDMS file, repeatedly\nwrite them to the IMU, until it is verified that they\narrived by comparing to a redundant IMU read."
        n125 = Build Array(u8 0 ("I2CRegister")) -> (w288:u8[])
        n126 = call <vilib>:"WPI_I2CWrite.vi"("I2CDataToSend"=w288, "I2CRegister"=u8 61 ("Data To Send hex 2"), "I2CDevRef"=w277) -> ("I2CDevRef"=w276:T1)  [unwired: 7 in, 1 out]
        n127 = Build Path(base path=path "u:/" ("file path (dialog if empty)"), name or relative path="Stored Cal File") -> (appended path=w273:path)
        n128 = TDMS Open(7:enum16{"1.0", "2.0"}."2.0" ("file format version (2.0)"), 10:T9."open (read-only)" ("operation (0:open)"), 11:w273) -> (3:w286:refnum<k34>)  [unwired: 4 in, 1 out]
        n129 = TDMS Read(0:w286, 5:"Cal" ("group name in (Untitled)"), 7:"Constants" ("channel name(s) in"), 12:u8[] []) -> (4:w287:refnum<k34>, 10:w275:u8[])  [unwired: 4 in, 4 out]
        n130 = while {
          tunnel: w275 -> [w297]
          tunnel: w276 -> [w302]
          tunnel: [w296] -> w274
          stop <- w293 stop-if-true
          n131 = for {
            N: 22 -> [_]
            tunnel: u8 85 ("Data To Send 2") -> [w317]
            tunnel: w297 -> [w315] mode=indexing
            tunnel: w302 -> [w316]
            tunnel: [w313] -> w299
            i -> [w318]
            n132 = Build Array(w315) -> (w314:u8[])
            n133 = Add(x=w317, y=w318) -> (x+y=w319:i32)
            n134 = call <vilib>:"WPI_I2CWrite.vi"("I2CDataToSend"=w314, "I2CRegister"=w319, "I2CDevRef"=w316) -> ("I2CDevRef"=w313:T1)  [unwired: 7 in, 1 out]
          }
          n135 = for {
            N: 22 -> [_]
            tunnel: u8 85 ("Data To Send 2") -> [w309]
            tunnel: [w308] -> w298 mode=concatenating
            tunnel: w299 -> [w307]
            tunnel: [w306] -> w296
            i -> [w305]
            n136 = Add(x=w309, y=w305) -> (x+y=w310:i32)
            n137 = Build Array(w310) -> (w311:i32[])
            n138 = call <vilib>:"WPI_I2CRead.vi"("I2CBytesToRead"=u8 1, "I2CRegister"=w311, "I2CDevRef"=w307) -> ("Data Out"=w308:u8[], "I2CDevRef"=w306:T1)  [unwired: 6 in, 1 out]
          }
          n139 = Equal?(x=w298, y=w297) -> (x = y?=w295:bool[])
          n140 = And Array Elements(Boolean array=w295) -> (logical AND=w293:bool)
          n141 = Wait (ms)(milliseconds to wait=u32 50) -> ()  [unwired: 1 out]
        }
        n142 = TDMS Close(11:w287) -> ()  [unwired: 1 in, 2 out]
        n143 = Build Array(w272) -> (w292:T10)
        n144 = call <vilib>:"WPI_I2CWrite.vi"("I2CDataToSend"=w292, "I2CRegister"=u8 61 ("Data To Send hex 2"), "I2CDevRef"=w274) -> ()  [unwired: 7 in, 2 out]
      }
      frame "Cal Status" {
        # "Poll the Cal_Status Register to indicate what the IMU reports regarding the calibration.\nContinue to update indicator for a set number of iterations to allow internal IMU Algo time to settle\nensuring IMU is ready for use once the IMUOpen operation has completed."
        n145 = while {
          tunnel: w322 -> [w333]
          i -> [w332]
          stop <- w330 stop-if-true
          n146 = Build Array(u8 53 ("Data To Send")) -> (w334:u8[])
          n147 = call <vilib>:"WPI_I2CRead.vi"("I2CBytesToRead"=u8 1, "I2CRegister"=w334, "I2CDevRef"=w333) -> ("Data Out"=w345:u8[])  [unwired: 6 in, 2 out]
          n148 = Greater Or Equal?(x=w332, y="Status delay") -> (x >= y?=w330:bool)
          n149 = Index Array(array=w345) -> (element=w344:u8)  [unwired: 1 in]
          n150 = Number To Boolean Array(number=w344) -> (Boolean array=w343:bool[])
          n151 = Index Array(array=w343) -> (element #1=w337:bool, element #2=w338:bool, element #3=w324:bool, element #4=w346:bool, element #5=w339:bool, element #6=w340:bool, element #7=w341:bool, element #8=w342:bool)  [unwired: 8 in]
          n152 = Wait (ms)(milliseconds to wait=u32 2 ("pre-cal wait")) -> ()  [unwired: 1 out]
          n153 = call "Status.vi"("Big"=w338, "Little"=w337) -> ("Cluster"=w329:T11)  [unwired: 2 in]
          n154 = call "Status.vi"("Big"=w346, "Little"=w324) -> ("Cluster"=w328:T11)  [unwired: 2 in]
          n155 = call "Status.vi"("Big"=w340, "Little"=w339) -> ("Cluster"=w327:T11)  [unwired: 2 in]
          n156 = call "Status.vi"("Big"=w342, "Little"=w341) -> ("Cluster"=w326:T11)  [unwired: 2 in]
          n157 = Bundle("Cluster"=w329, "Cluster"=w328, "Cluster"=w327, "Cluster"=w326) -> (→"Cal Status":T4)  [unwired: 1 in]
        }
      }
      frame "Idle" {
        n158 = case shown="True" w350 {
          tunnel: [TRUE w355] -> w349
          tunnel: w348 -> [_ w352]
          frame False {
          }
          frame True {
            w358 = "\n"
            n159 = Concatenate Strings(w358, w358) -> (w354:string)
            n160 = Concatenate Strings("Your BNO055 calibration constants\nare stored in this file:" ("message"), w354, w352, w354, "Click OK when you have recorded the filename,\nthen stop the code, set Calibrate? to FALSE,\nand provide this filename to the\nIMUOrientOpen subVI \"Stored Cal File\" terminal." ("string"), w354, "When you next run IMUOrientOpen,\nthese calibration constants will be\nautomatically loaded and the IMU\nwill be ready for use upon startup." ("string"), w354, "The RoboBees Team 836 ... Orient to STEM!" ("string")) -> (w360:string)
            n161 = feedback #3(FALSE ("true")) -> (w362:bool)
            n162 = case shown="False" w362 {
              selector: w362 -> [_ w365]
              tunnel: [w364 w365] -> w355
              tunnel: w360 -> [w363 _]
              frame False {
                n163 = One Button Dialog(message=w363) -> (true=w364:bool)  [unwired: 1 in]
              }
              frame True {
              }
            }
            n164 = feedback-in #3(w355) -> ()
          }
        }
      }
    }
    n165 = local read "Bad result"() -> (w19:bool)
    "Setup ct" <- w25
    "Setup State" <- w13
  }
  "I2CDevRef" <- w7
  "Bad result" <- w4
